vi "Update Map.vi"(0 "Pose in Radians":dbl, 1 "Y":dbl, 2 "X":dbl) -> ()   [LabVIEW 2010]
uses:
  Main Global.vi
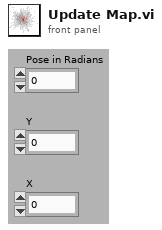
[diagram p1: front panel]
types:
  T1 = typedef "Streaming Data.ctl" = cluster{"Bump Right":bool, "Bump Left":bool, "Wheel Drop Right":bool, "Wheel Drop Left":bool, "Wheel Drop Caster":bool, "Wall":bool, "Cliff Left":bool, "Cliff Front Left":bool, "Cliff Front Right":bool, "Cliff Right":bool, "IR Red":bool, "IR Green":bool, "IR Force":bool, "Play":bool, "Advance":bool, "Battery Charge":i16}
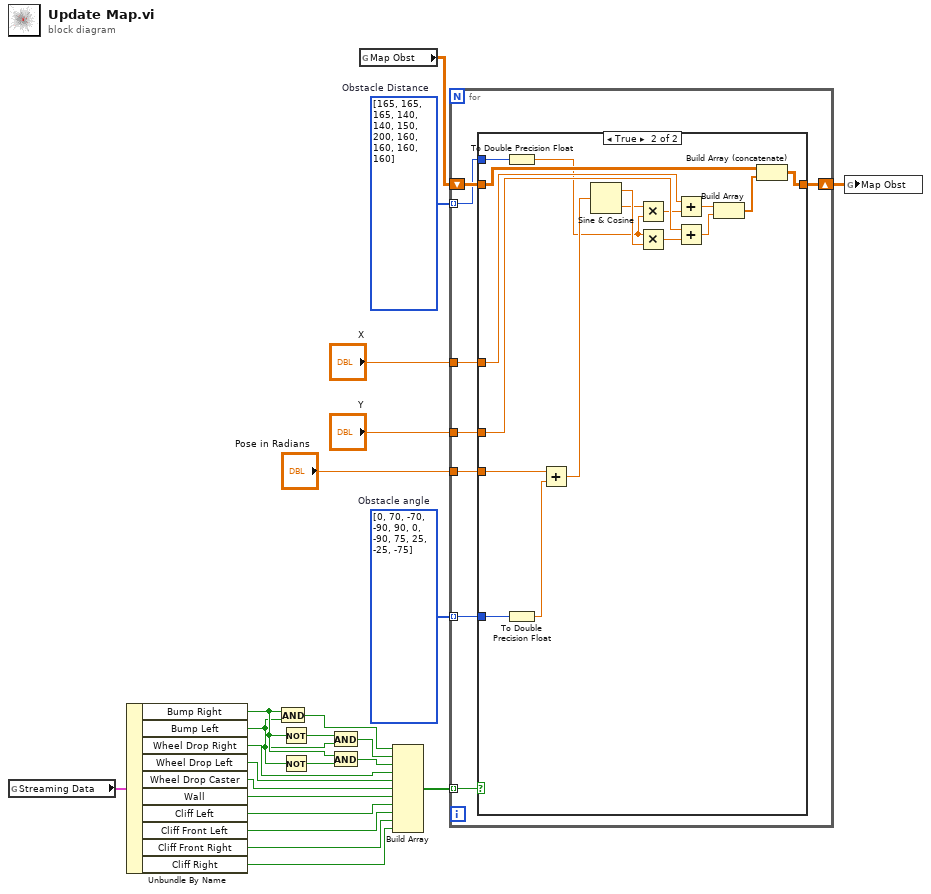
[diagram p0: block diagram]
diagram:
  w17 = i32[] [0, 70, -70, -90, 90, 0, -90, 75, 25, -25, -75]  # Obstacle angle
  w18 = i32[] [165, 165, 165, 140, 140, 150, 200, 160, 160, 160, 160]  # Obstacle Distance
  n1 = global read "Main Global.vi" "Streaming Data"() -> (w1:T1)
  n2 = Unbundle By Name(w1) -> ("Bump Right"=w13:bool, "Bump Left"=w11:bool, "Wheel Drop Right"=w2:bool, "Wheel Drop Left"=w3:bool, "Wheel Drop Caster"=w4:bool, "Wall"=w5:bool, "Cliff Left"=w6:bool, "Cliff Front Left"=w7:bool, "Cliff Front Right"=w8:bool, "Cliff Right"=w9:bool)
  n3 = And(x=w13, y=w11) -> (x .and. y?=w14:bool)
  n4 = Not(x=w13) -> (.not. x?=w10:bool)
  n5 = Not(x=w11) -> (.not. x?=w12:bool)
  n6 = And(x=w10, y=w11) -> (x .and. y?=w15:bool)
  n7 = And(x=w13, y=w12) -> (x .and. y?=w16:bool)
  n8 = global read "Main Global.vi" "Map Obst"() -> (w20:dbl[][])
  n9 = Build Array(w14, w15, w16, w2, w3, w4, w5, w6, w7, w8, w9) -> (w19:bool[])
  n10 = for {
    tunnel: w17 -> [w27] mode=indexing
    tunnel: w18 -> [w25] mode=indexing
    tunnel: w19 -> [w32] mode=indexing
    shift-right: [w30] -> w24
    shift-left: w20 -> [w31]
    tunnel: "X" -> [w29]
    tunnel: "Y" -> [w28]
    tunnel: "Pose in Radians" -> [w26]
    n11 = case shown="True" w32 {
      tunnel: w31 -> [w33 w50]
      tunnel: [w33 w49] -> w30
      tunnel: w29 -> [_ w48]
      tunnel: w28 -> [_ w47]
      tunnel: w27 -> [_ w45]
      tunnel: w26 -> [_ w43]
      tunnel: w25 -> [_ w39]
      frame False {
      }
      frame True {
        n12 = To Double Precision Float(number=w39) -> (double precision float=w38:dbl)
        n13 = To Double Precision Float(number=w45) -> (double precision float=w44:dbl)
        n14 = Add(x=w43, y=w44) -> (x+y=w42:dbl)
        n15 = Sine & Cosine(0:w42) -> (1:w41:dbl, 2:w40:dbl)
        n16 = Multiply(x=w40, y=w38) -> (x*y=w34:dbl)
        n17 = Multiply(x=w38, y=w41) -> (x*y=w36:dbl)
        n18 = Add(x=w48, y=w34) -> (x+y=w35:dbl)
        n19 = Add(x=w47, y=w36) -> (x+y=w37:dbl)
        n20 = Build Array(w35, w37) -> (w46:dbl[])
        n21 = Build Array (concatenate)(w50, w46) -> (w49:dbl[][])
      }
    }
  }
  n22 = global write "Main Global.vi" "Map Obst"(w24) -> ()
